vi "Convert V to Rt - DBL.vi"(7 "ThermConfig":T1, 9 "Vmeas":dbl caption="Measured Voltage", 10 "Rref":dbl caption="Reference Resistance", 11 "Vsource":dbl caption="Source Voltage") -> (3 "Rt":dbl)   [LabVIEW 2014, in "Temperature.lvlib"]
doc: "Convert a voltage registered by a thermistor circuit to a thermistor resistance using the equation for a voltage divider. The thermistor resistance can then be readily converted to a temperature using the <B>Steinhart-Hart </b> equations. The <b>ThermConfig</b> (bottom, top) refers to the position of the thermistor in the voltage divider circuit. If the thermistor is located nearest ground, the config is Bottom."
uses:
  Temperature.lvlib
  Thermistor Position.ctl
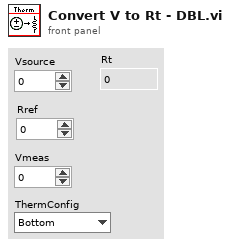
[diagram p1: front panel]
types:
  T1 = typedef "Temperature.lvlib/Thermistor Position.ctl" = enum8{"Bottom", "Top"}
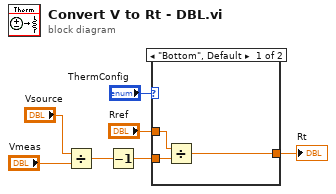
[diagram p0: block diagram]
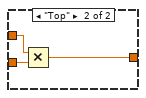
[diagram p2: hidden frame]
diagram:
  n1 = Divide(x="Vsource", y="Vmeas") -> (x/y=w6:dbl)
  n2 = Decrement(x=w6) -> (x-1=w4:dbl)
  n3 = case shown="\"Bottom\", Default" "ThermConfig" {
    tunnel: w4 -> [w9 w13]
    tunnel: [w8 w12] -> w1
    tunnel: "Rref" -> [w10 w11]
    frame "Bottom", Default {
      n4 = Divide(x=w10, y=w9) -> (x/y=w8:dbl)
    }
    frame "Top" {
      n5 = Multiply(x=w11, y=w13) -> (x*y=w12:dbl)
    }
  }
  "Rt" <- w1
